vi "Start.vi"(8 "error in (no error)":errorcluster, 10 "Message in":refnum<class "StartMessage.lvclass">, 11 "Tomo in":refnum<class "Tomo.lvclass">) -> (0 "error out":errorcluster, 3 "Tomo out":refnum<class "Tomo.lvclass">)   [LabVIEW 2012, in "Tomo.lvclass"]
doc: "This member function is called when the statemachine in the run.vi receives an 'start' command. It relays the message to all observers of the component.\n\nOverride this member function in your derived class if you need additional start functionality (but don't forget to call the parent method)."
uses:
  Tomo.lvclass
  <vilib>/Distrio/Murmex/StartMessage/StartMessage.lvclass
  <vilib>/Distrio/Murmex/Murmex/Murmex.lvclass
  <vilib>/Distrio/Murmex/GenericMessage/GenericMessage.lvclass
panel:
  # "This member function is called when the statemachine in the run.vi receives an 'start' command. It relays the message to all observers of the component.\n\nOverride this member function in your derived class if you need additional start functionality (but don't forget to call the parent method)."
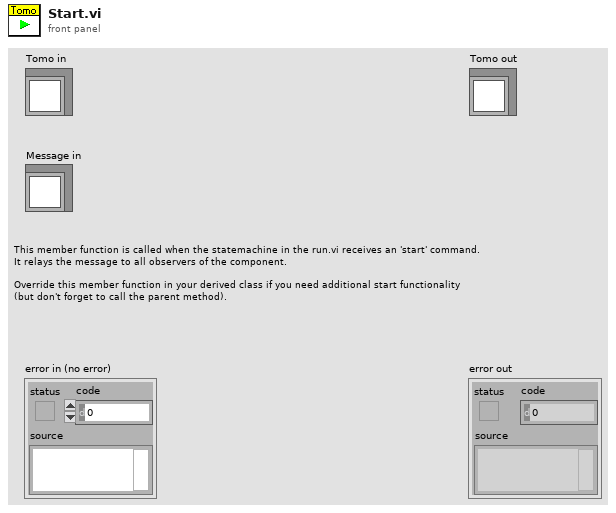
[diagram p1: front panel]
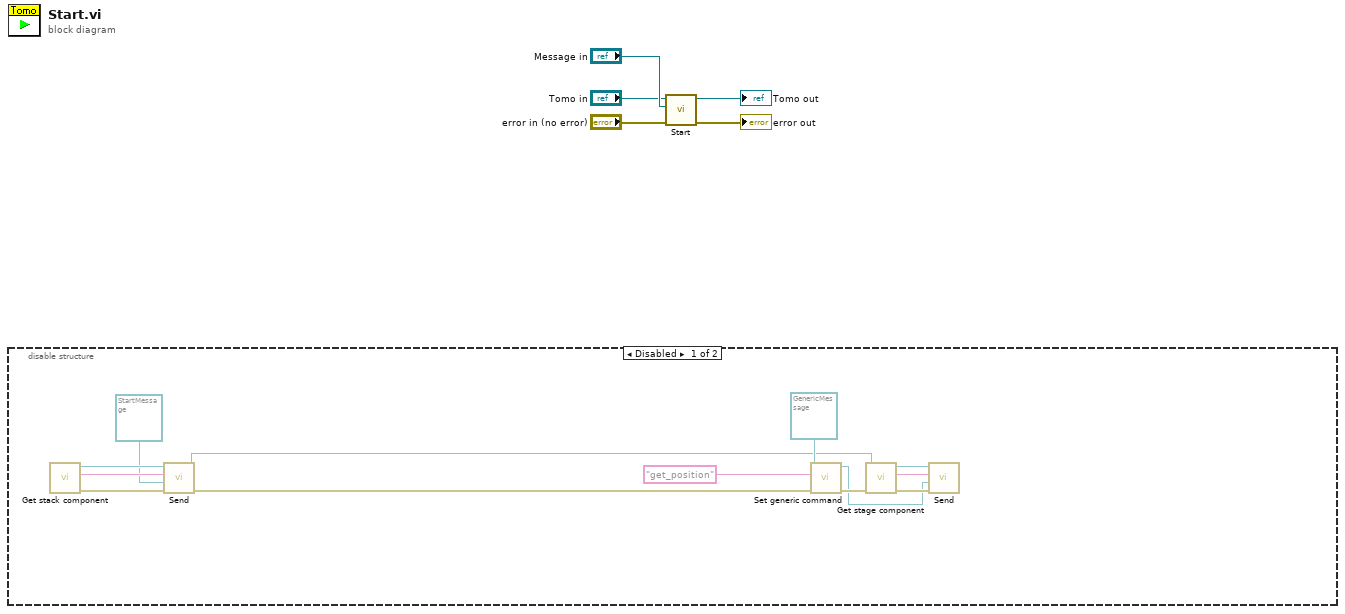
[diagram p0: block diagram]
diagram:
  n1 = disable-structure shown="Disabled" {
    frame Disabled {
      n2 = call-dynamic "Get stack component.vi"() -> ("error out"=w11:errorcluster, "stack component"=w9:string, "Tomo out"=w10:refnum<class "Tomo.lvclass">)  [unwired: 9 in]
      n3 = call <vilib>:"Send.vi"("error in (no error)"=w11, "Message"=refnum<class "StartMessage.lvclass"> refnum ("Message in"), "recipient"=w9, "Murmex in"=w10) -> ("error out"=w8:errorcluster, "Murmex out"=w7:refnum<class "Tomo.lvclass">)  [unwired: 6 in]
      n4 = call <vilib>:"Set generic command.vi"("error in (no error)"=w8, "generic command"="get_position", "GenericMessage in"=refnum<class "GenericMessage.lvclass"> refnum ("Message in")) -> ("error out"=w17:errorcluster, "GenericMessage out"=w13:refnum<class "GenericMessage.lvclass">)  [unwired: 7 in]
      n5 = call-dynamic "Get stage component.vi"("error in (no error)"=w17, "Tomo in"=w7) -> ("error out"=w16:errorcluster, "stage component"=w14:string, "Tomo out"=w15:refnum<class "Tomo.lvclass">)  [unwired: 7 in]
      n6 = call <vilib>:"Send.vi"("error in (no error)"=w16, "Message"=w13, "recipient"=w14, "Murmex in"=w15) -> ()  [unwired: 6 in, 2 out]
    }
    frame Enabled {
    }
  }
  n7 = call-parent "Start.vi"("error in (no error)"="error in (no error)", "Message in"="Message in", "Murmex in"="Tomo in") -> ("error out"=→"error out":errorcluster, "Murmex out"=→"Tomo out":refnum<class "Tomo.lvclass">)  [unwired: 7 in]
